vi "GetColor.vi"(8 "error in (no error)":errorcluster, 11 "ColorRGB in":refnum<class "ColorCMYK.lvclass">) -> (0 "error out":errorcluster, 2 "Color":u32(colorbox), 3 "ColorRGB out":refnum<class "ColorCMYK.lvclass">)   [LabVIEW 2021, in "Picture2D.lvlib" / "ColorCMYK.lvclass"]
uses:
  ColorCMYK.lvclass
  ColorCMYK.lvclass/ColorCMYK.ctl
  Color/Color.lvclass
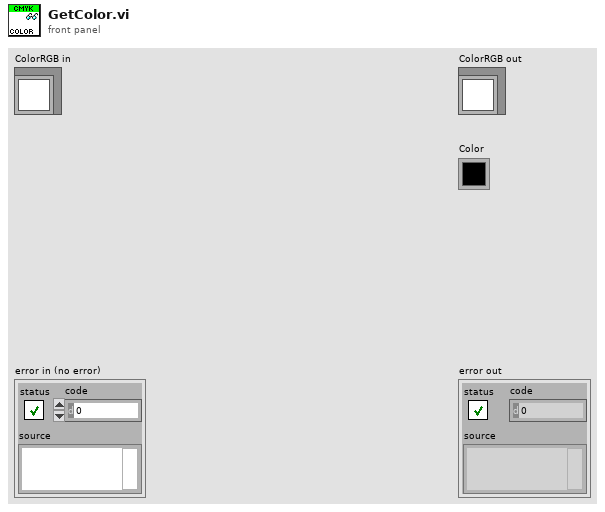
[diagram p1: front panel]
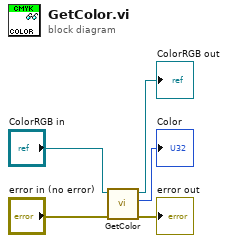
[diagram p0: block diagram]
diagram:
  n1 = call-parent "GetColor.vi"("error in (no error)"="error in (no error)", "Color in"="ColorRGB in") -> ("error out"=→"error out":errorcluster, "Color"=→"Color":u32, "Color out"=→"ColorRGB out":refnum<class "ColorCMYK.lvclass">)  [unwired: 7 in]
